vi "LIA.SR810.ReftoDVR.vi"(10 "Ref":u32 format="%08x") -> (2 "Ref":T1)   [LabVIEW 2017, in "LIA.SR810.lvclass"]
doc: "JKI State Machine Objects (SMO) 1.0.0.5\nJKI - JKI\nCopyright (c) 2016, JKI"
uses:
  LIA.SR810.lvclass
  Typedefs/Configuration--Cluster.ctl
  Typedefs/DataChanged--EventData--Cluster.ctl
  Typedefs/PublicEvents--Cluster.ctl
  Typedefs/API Inputs--Cluster.ctl
  Typedefs/ProtectedEvents--Cluster.ctl
  Typedefs/PrivateData--Cluster.ctl
  Typedefs/PrivateData--Ref.ctl
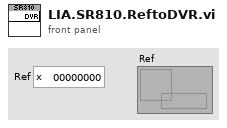
[diagram p1: front panel]
types:
  T1 = typedef "LIA.SR810.lvclass/PrivateData--Ref.ctl" = refnum<data-value>
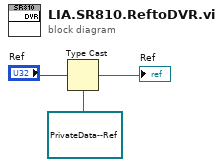
[diagram p0: block diagram]
diagram:
  n1 = Type Cast(type=T1 refnum ("Ref"), x="Ref") -> (*(type *) &x=→"Ref":T1)
